vi "3-1.vi"() -> ()   [LabVIEW 2017]
panel:
  out "余弦":dbl
  out "正弦":dbl
  in  "x":dbl
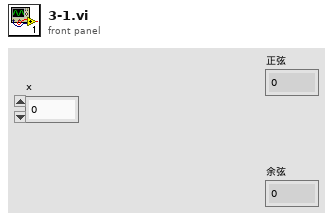
[diagram p1: front panel]
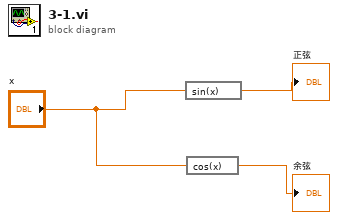
[diagram p0: block diagram]
diagram:
  n1 = expression code="sin(x)"("x") -> (→"正弦":dbl)
  n2 = expression code="cos(x)"("x") -> (→"余弦":dbl)
